vi "Unbenannt 1.vi"() -> ()   [LabVIEW 2017]
panel:
  out "Ausgabe-String":string
  out "Erstes Zeichen zuletzt":string
  in  "zu Einrichtung Basis":u8=3 min=2
  in  "Basis":i8=3 min=2 max=16
  in  "Zahl":string
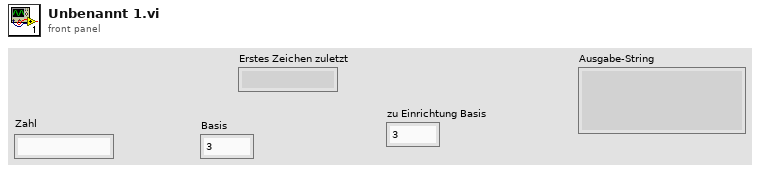
[diagram p1: front panel]
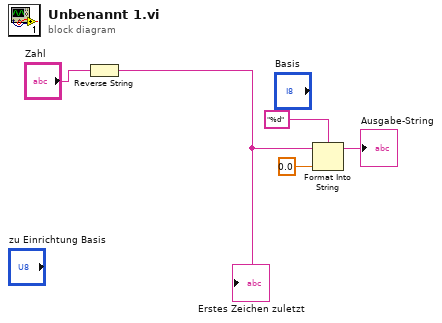
[diagram p0: block diagram]
diagram:
  n1 = Reverse String(1:"Zahl") -> (0:w4:string)
  "Erstes Zeichen zuletzt" <- w4
  n2 = Format Into String(format string="%d" ("Format-String"), initial string=w4, 0.0 ("Eingang 1")) -> (resulting string=→"Ausgabe-String":string)  [unwired: 1 in, 1 out]
